vi "界面0-硬件配置.vi"() -> ()   [LabVIEW 2013]
uses:
  <vilib>/Utility/config.llb/Read Key (I32).vi
  <vilib>/Utility/config.llb/NI_LVConfig.lvlib
panel:
  out "Boolean":bool
  in  "项目->":bool
  in  "工控机配置":bool
  in  "伺服卡配置":bool
  # "欢迎使用\n                  \n\n\n油动机试验系统\n\n  上海电气电站设备有限公司"
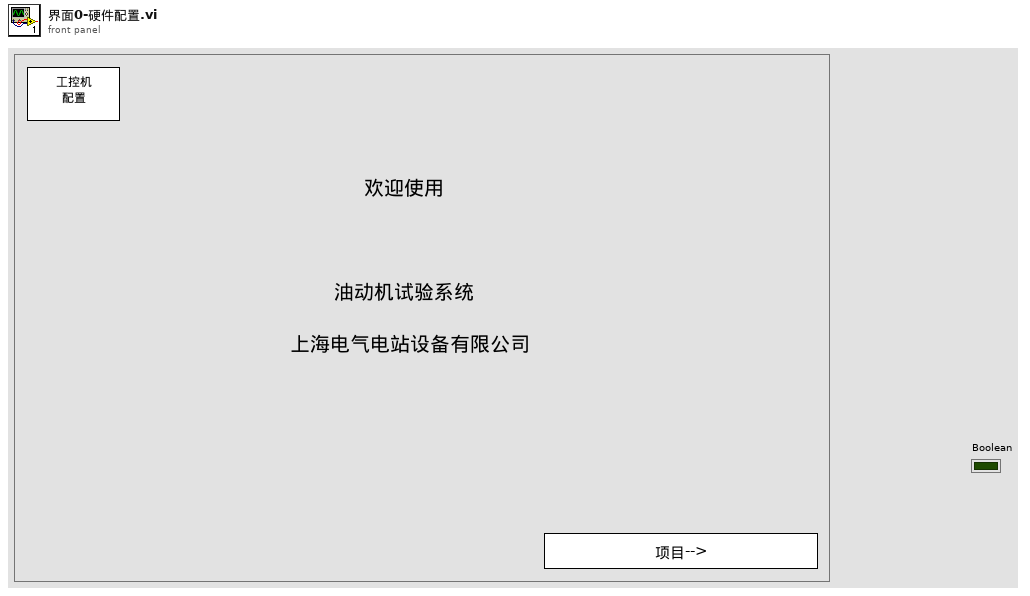
[diagram p1: front panel]
types:
  T1 = typedef "NI_LVConfig.lvlib/Config Data RefNum.ctl" = refnum<k1>
  T2 = enum32{"Bad", "Idle", "Run top level", "Running"}
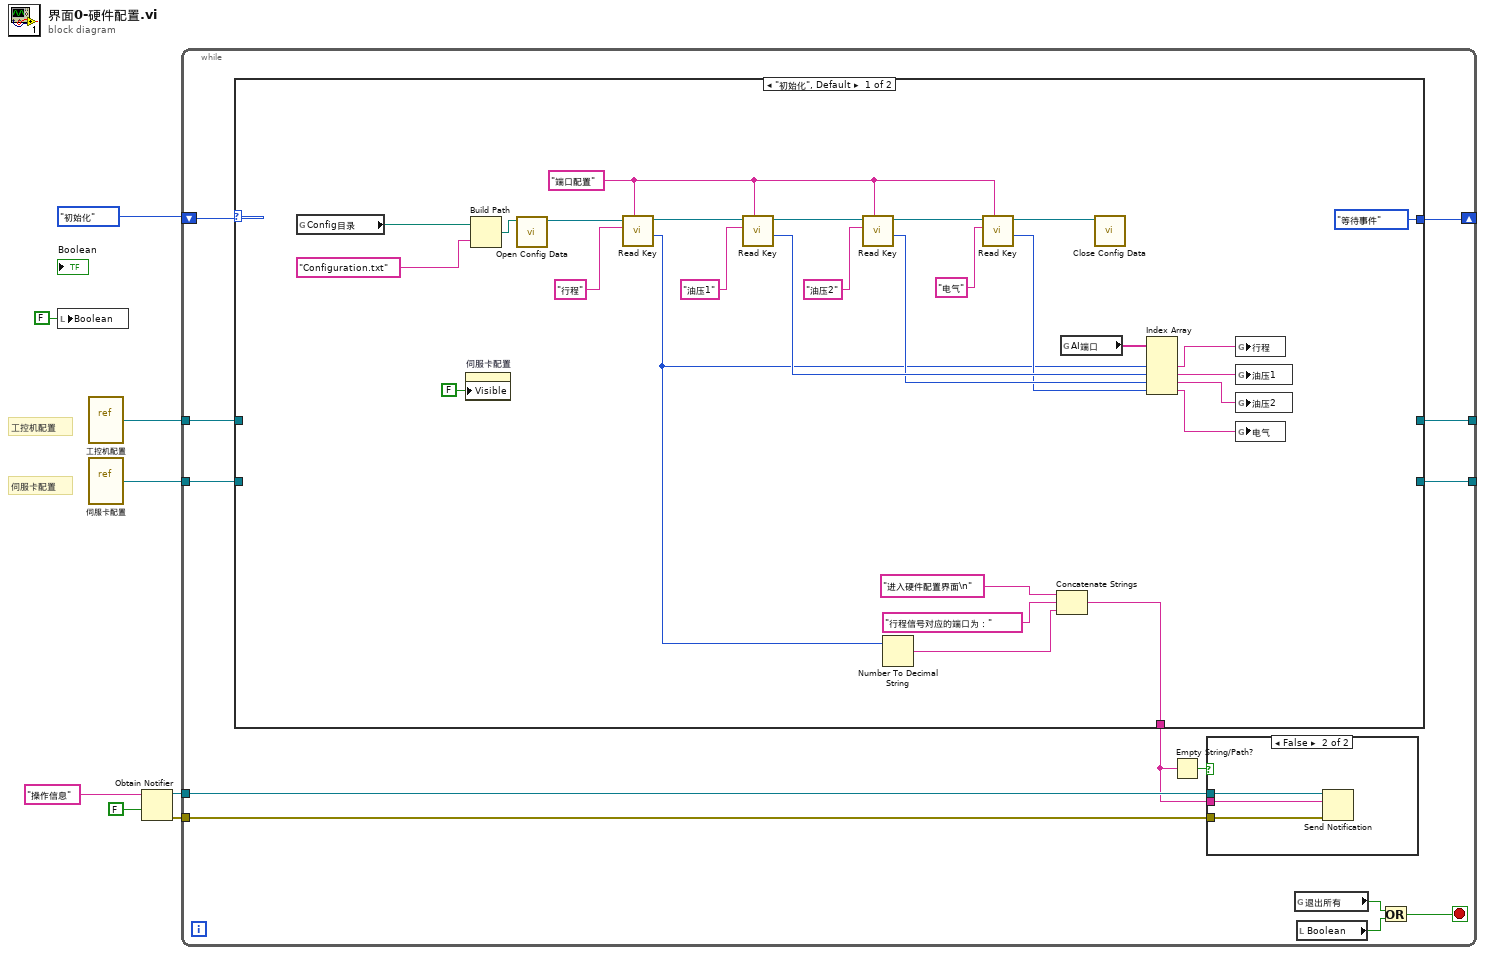
[diagram p0: block diagram]
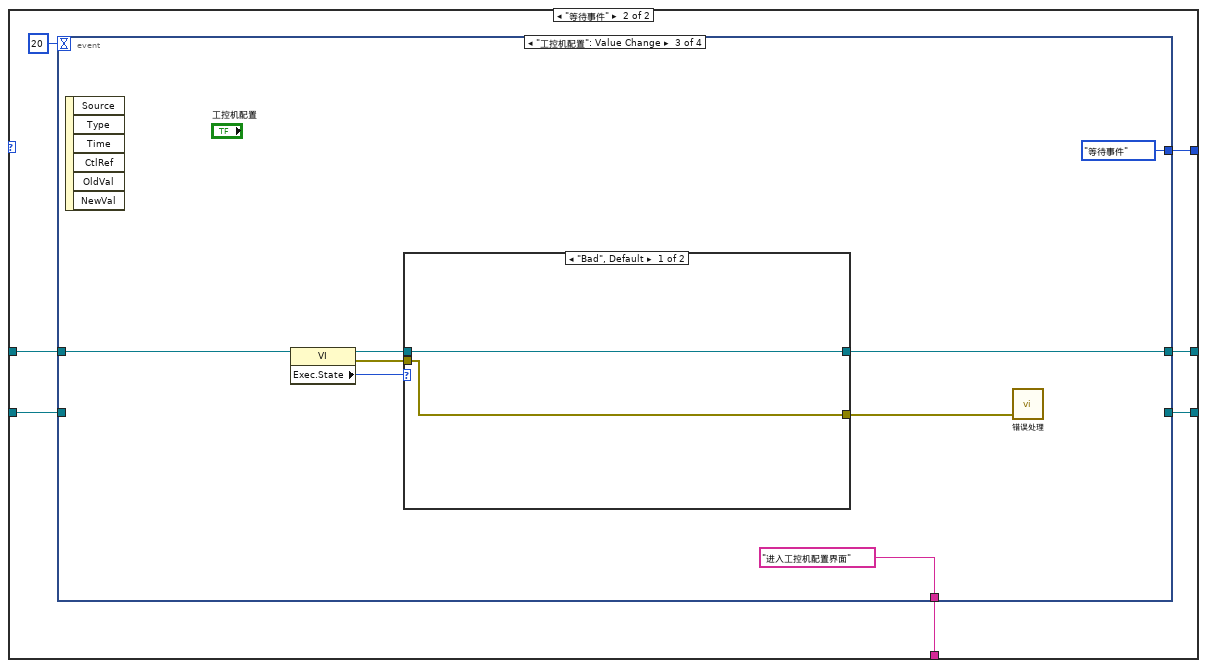
[diagram p3: hidden frame]
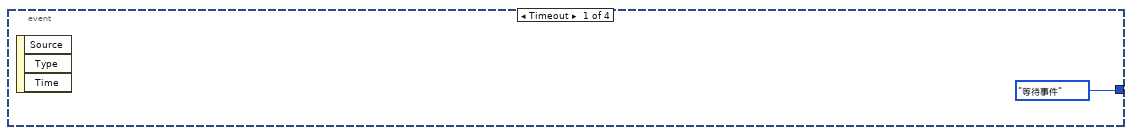
[diagram p4: hidden frame]
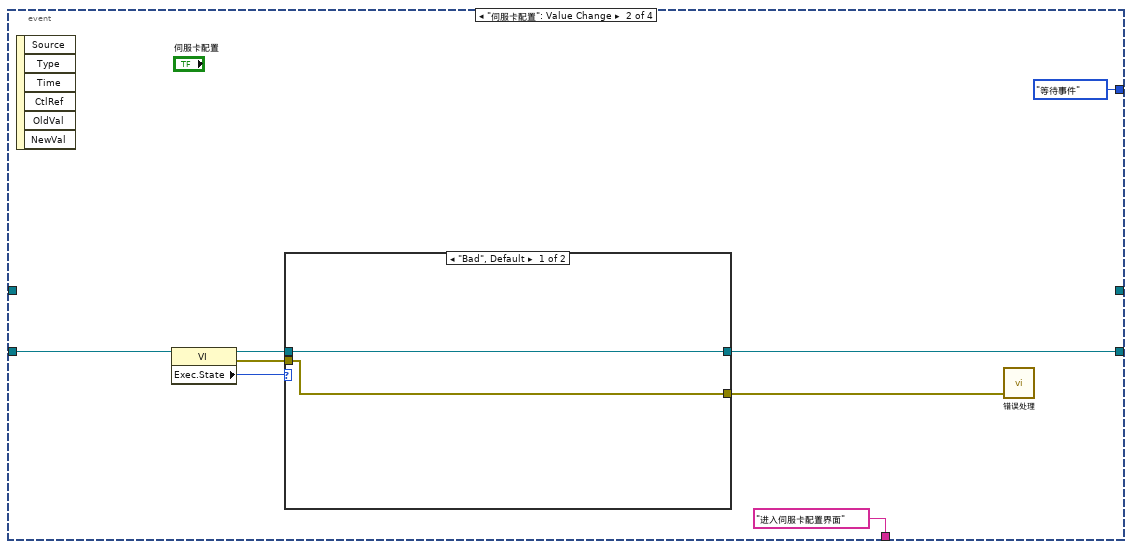
[diagram p5: hidden frame]
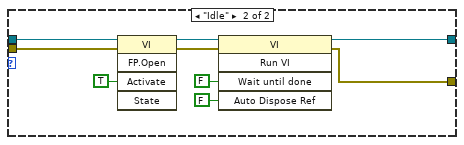
[diagram p6: hidden frame]
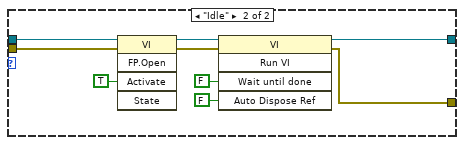
[diagram p7: hidden frame]
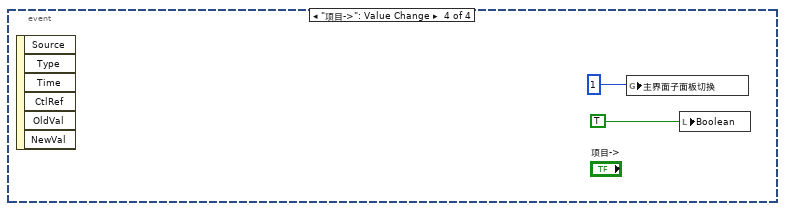
[diagram p8: hidden frame]
diagram:
  w6 = "操作信息"
  # "伺服卡配置"
  # "工控机配置"
  n1 = local write "Boolean"(FALSE ("Boolean")) -> ()
  n2 = vi-ref "工控机配置.vi"() -> (w2:refnum<vi>)
  n3 = vi-ref "伺服卡配置.vi"() -> (w1:refnum<vi>)
  n4 = Obtain Notifier(name (unnamed)=w6, notification data type=w6, create if not found? (T)=FALSE) -> (notifier out=w5:refnum<notifier>, error out=w4:errorcluster)  [unwired: 1 in, 1 out]
  n5 = while {
    shift-right: [w20] -> _
    shift-left: enum16{"初始化", "等待事件", "退出"}."初始化" -> [w21]
    tunnel: w5 -> [w16]
    tunnel: w4 -> [w15]
    tunnel: w2 -> [w12]
    tunnel: [w11] -> _
    tunnel: w1 -> [w10]
    tunnel: [w9] -> _
    stop <- w17 stop-if-true
    n6 = case shown="\"初始化\", Default" w21 {
      tunnel: [w29 w59] -> w14
      tunnel: [enum16{"初始化", "等待事件", "退出"}."等待事件" w58] -> w20
      tunnel: w12 -> [_ w56]
      tunnel: [_ w55] -> w11
      tunnel: w10 -> [_ w54]
      tunnel: [_ w53] -> w9
      frame "初始化", Default {
        w47 = "端口配置" ("Section")
        n7 = global read "Config目录.vi" "Config目录"() -> (w43:path)
        n8 = property on="伺服卡配置" class="Bool"("Visible"=FALSE) -> ()  [unwired: 2 in, 2 out]
        n9 = Build Path(base path=w43, name or relative path="Configuration.txt") -> (appended path=w41:path)
        n10 = call <vilib>:"Open Config Data.vi"("configuration file path"=w41) -> ("refnum"=w40:T1)  [unwired: 8 in, 2 out]
        n11 = call-poly <vilib>:"Read Key.vi"("section"=w47, "key"="行程" ("Key"), "refnum"=w40) -> ("value"=w33:i32, "refnum out"=w50:T1)  [unwired: 5 in, 2 out]
        n12 = call-poly <vilib>:"Read Key.vi"("section"=w47, "key"="油压1" ("Key"), "refnum"=w50) -> ("value"=w36:i32, "refnum out"=w49:T1)  [unwired: 5 in, 2 out]
        n13 = call-poly <vilib>:"Read Key.vi"("section"=w47, "key"="油压2" ("Key"), "refnum"=w49) -> ("value"=w35:i32, "refnum out"=w48:T1)  [unwired: 5 in, 2 out]
        n14 = Number To Decimal String(number=w33) -> (decimal integer string=w30:string)  [unwired: 1 in]
        n15 = call-poly <vilib>:"Read Key.vi"("section"=w47, "key"="电气" ("Key"), "refnum"=w48) -> ("value"=w34:i32, "refnum out"=w39:T1)  [unwired: 5 in, 2 out]
        n16 = Concatenate Strings("进入硬件配置界面\n", "行程信号对应的端口为：", w30) -> (w29:string)
        n17 = global read "AI端口.vi" "AI端口"() -> (w38:tag[])
        n18 = call <vilib>:"Close Config Data.vi"("refnum"=w39) -> ()  [unwired: 9 in, 2 out]
        n19 = Index Array(array=w38, index #2=w33, index #3=w36, index #4=w35, index #5=w34) -> (element #2=w37:tag, element #3=w27:tag, element #4=w26:tag, element #5=w25:tag)  [unwired: 1 in, 1 out]
        n20 = global write "AI端口_行程.vi" "行程"(w37) -> ()
        n21 = global write "AI端口_油压1.vi" "油压1"(w27) -> ()
        n22 = global write "AI端口_油压2.vi" "油压2"(w26) -> ()
        n23 = global write "AI端口_电气.vi" "电气"(w25) -> ()
      }
      frame "等待事件" {
        n24 = event shown="[2] \"工控机配置\": Value Change" {
          selector: _ -> [_ _ _ _]
          dyn-events: _ -> [_ _ _ _]
          timeout: 20 -> [_ _ _ _]
          tunnel: [_ "进入伺服卡配置界面" "进入工控机配置界面" _] -> w59
          tunnel: [enum16{"初始化", "等待事件", "退出"}."等待事件" enum16{"初始化", "等待事件", "退出"}."等待事件" enum16{"初始化", "等待事件", "退出"}."等待事件" _] -> w58
          tunnel: w56 -> [_ _ w86 _]
          tunnel: [_ _ w83 _] -> w55
          tunnel: w54 -> [_ w64 _ _]
          tunnel: [_ w63 _ _] -> w53
          event Timeout {
            n25 = event-data() -> ()  [unwired: 1 in, 3 out]
          }
          event "伺服卡配置": Value Change {
            n26 = event-data() -> ()  [unwired: 1 in, 6 out]
            n27 = property class="VI"(reference=w64) -> (reference out=w65:refnum<vi>, error out=w62:errorcluster, "Exec.State"=w66:T2)  [unwired: 1 in]
            n28 = case shown="\"Bad\", Default" w66 {
              tunnel: w65 -> [w70 w78]
              tunnel: [w70 w74] -> w63
              tunnel: w62 -> [w69 w73]
              tunnel: [w69 w71] -> w61
              frame "Bad", Default {
              }
              frame "Idle" {
                n29 = invoke class="VI" method="FP.Open"(reference=w78, error in=w73, "Activate"=TRUE ("Activate?")) -> (reference out=w76:refnum<vi>, error out=w72:errorcluster)  [unwired: 2 in, 3 out]
                n30 = invoke class="VI" method="Run VI"(reference=w76, error in=w72, "Wait until done"=FALSE ("Wait Until Done"), "Auto Dispose Ref"=FALSE ("Auto Dispose Reference")) -> (reference out=w74:refnum<vi>, error out=w71:errorcluster)  [unwired: 1 in, 3 out]
              }
            }
            n31 = call "错误处理.vi"("error in (no error)"=w61) -> ()  [unwired: 2 in]
          }
          event "工控机配置": Value Change {
            n32 = event-data() -> ()  [unwired: 1 in, 6 out]
            n33 = property class="VI"(reference=w86) -> (reference out=w84:refnum<vi>, error out=w81:errorcluster, "Exec.State"=w85:T2)  [unwired: 1 in]
            n34 = case shown="\"Bad\", Default" w85 {
              tunnel: w84 -> [w89 w97]
              tunnel: [w89 w93] -> w83
              tunnel: w81 -> [w88 w92]
              tunnel: [w88 w90] -> w80
              frame "Bad", Default {
              }
              frame "Idle" {
                n35 = invoke class="VI" method="FP.Open"(reference=w97, error in=w92, "Activate"=TRUE ("Activate?")) -> (reference out=w95:refnum<vi>, error out=w91:errorcluster)  [unwired: 2 in, 3 out]
                n36 = invoke class="VI" method="Run VI"(reference=w95, error in=w91, "Wait until done"=FALSE ("Wait Until Done"), "Auto Dispose Ref"=FALSE ("Auto Dispose Reference")) -> (reference out=w93:refnum<vi>, error out=w90:errorcluster)  [unwired: 1 in, 3 out]
              }
            }
            n37 = call "错误处理.vi"("error in (no error)"=w80) -> ()  [unwired: 2 in]
          }
          event "项目->": Value Change {
            n38 = event-data() -> ()  [unwired: 1 in, 6 out]
            n39 = global write "主界面子面板切换.vi" "主界面子面板切换"(1) -> ()
            n40 = local write "Boolean"(TRUE ("Boolean")) -> ()
          }
        }
      }
    }
    n41 = Empty String/Path?(string/path=w14) -> (empty?=w13:bool)
    n42 = case shown="False" w13 {
      tunnel: w16 -> [_ w24]
      tunnel: w15 -> [_ w23]
      tunnel: w14 -> [_ w22]
      frame True {
      }
      frame False {
        n43 = Send Notification(notification=w22, notifier=w24, error in (no error)=w23) -> ()  [unwired: 2 out]
      }
    }
    n44 = global read "退出所有.vi" "退出所有"() -> (w19:bool)
    n45 = local read "Boolean"() -> (w18:bool)
    n46 = Or(x=w19, y=w18) -> (x .or. y?=w17:bool)
  }
